vi "SaveConfigFile.vi"(0 "error in (no error)":errorcluster, 1 "IP":string caption="Robot IP Address", 2 "Licensee":string, 3 "Key":string) -> (20 "error out":errorcluster)   [LabVIEW 2016]
uses:
  <vilib>/Utility/config.llb/NI_LVConfig.lvlib
  <vilib>/Utility/config.llb/Write Key (String).vi
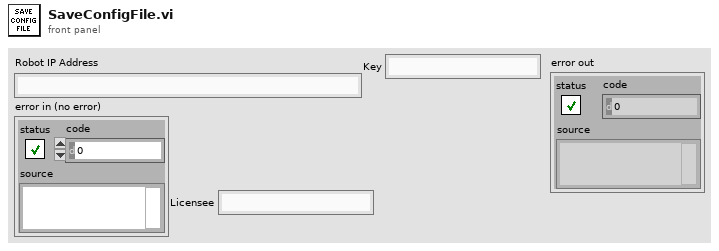
[diagram p1: front panel]
types:
  T1 = typedef "NI_LVConfig.lvlib/Config Data RefNum.ctl" = refnum<k1>
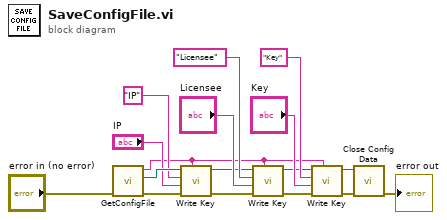
[diagram p0: block diagram]
diagram:
  n1 = call "GetConfigFile.vi"("error in (no error)"="error in (no error)") -> ("error out"=w16:errorcluster, "refnum"=w15:T1, "section"=w3:string)  [unwired: 8 in]
  n2 = call-poly <vilib>:"Write Key.vi"("section"=w3, "error in (no error)"=w16, "value"="IP", "key"="IP", "refnum"=w15) -> ("error out"=w1:errorcluster, "refnum out"=w2:T1)  [unwired: 4 in, 1 out]
  n3 = call-poly <vilib>:"Write Key.vi"("section"=w3, "error in (no error)"=w1, "value"="Licensee", "key"="Licensee", "refnum"=w2) -> ("error out"=w6:errorcluster, "refnum out"=w7:T1)  [unwired: 4 in, 1 out]
  n4 = call-poly <vilib>:"Write Key.vi"("section"=w3, "error in (no error)"=w6, "value"="Key", "key"="Key", "refnum"=w7) -> ("error out"=w5:errorcluster, "refnum out"=w8:T1)  [unwired: 4 in, 1 out]
  n5 = call <vilib>:"Close Config Data.vi"("error in (no error)"=w5, "refnum"=w8) -> ("error out"=→"error out":errorcluster)  [unwired: 8 in, 1 out]
